vi "Harv_2_9.vi"(0 "HarvSetpoints":dbl[](array[numeric]), 1 "HarvPot":dbl, 3 "Count":i32, 4 "BallAcquired":bool, 5 "FireBallSen":bool, 6 "Fire":bool, 7 "Harvest":bool, 8 "HPButton":bool, 9 "inAuton?":bool, 10 "WinchDown":bool, 11 "AutonMoved":bool, 12 "HarvPivUP":bool, 13 "HarvPivPickupLim":bool) -> (14 "HarvPower":dbl, 15 "HarvRoller":dbl, 16 "AutonReadyToMove":bool, 17 "CountOut":i32, 18 "HarvStart":bool, 19 "HarvCleared":bool)   [LabVIEW 2013]
panel:
  in  "MotorScale":dbl=1.5
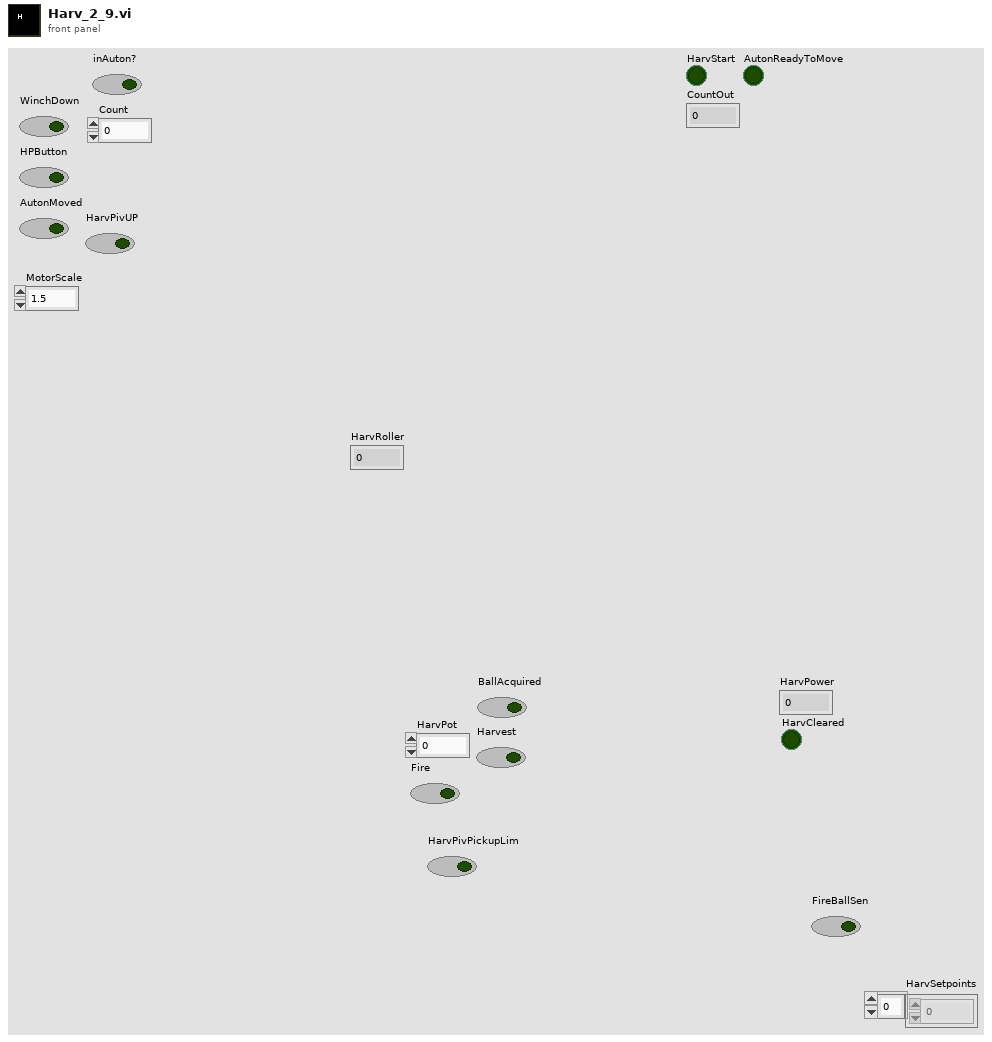
[diagram p1: front panel]
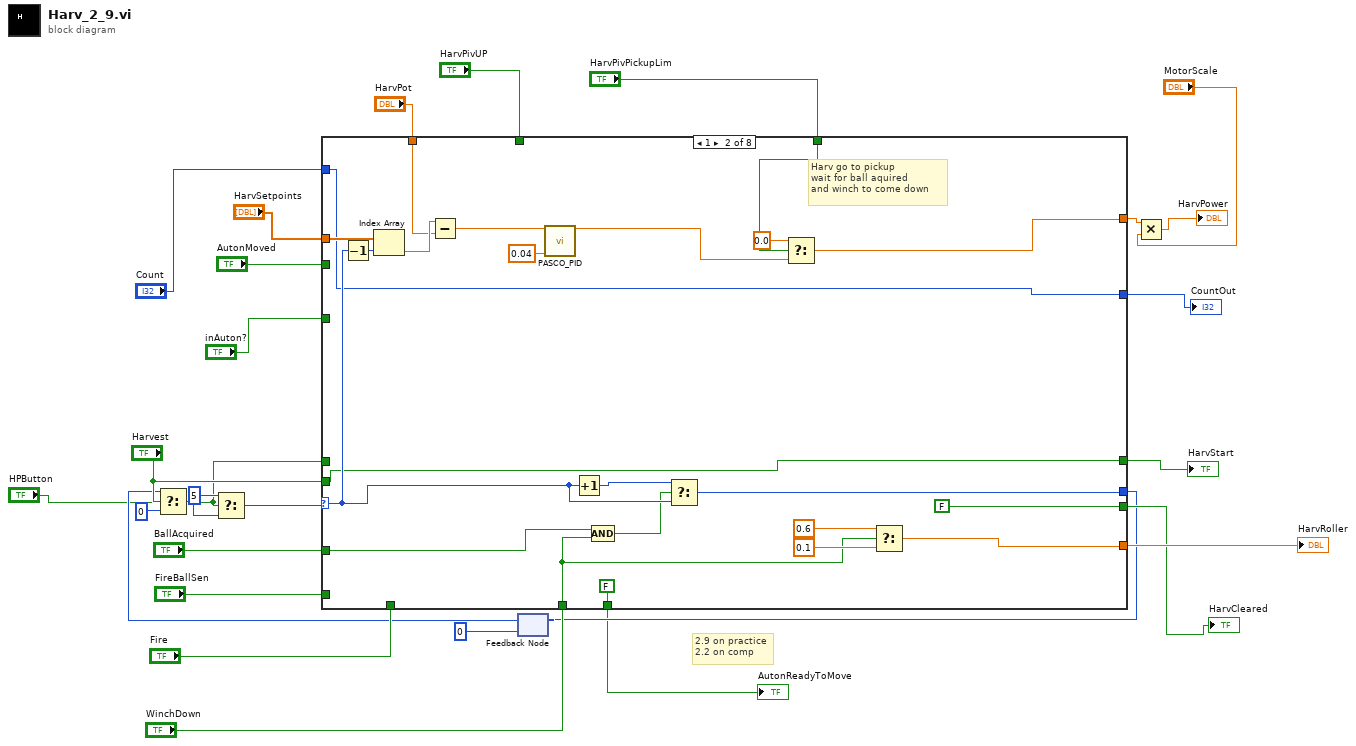
[diagram p0: block diagram]
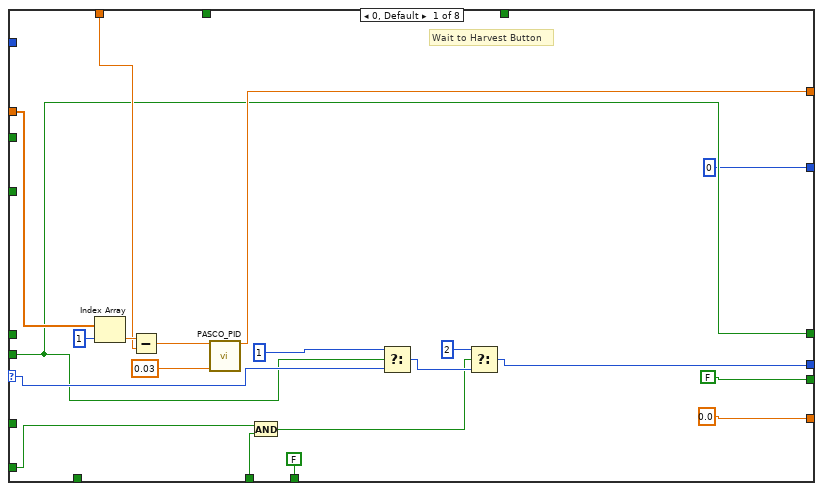
[diagram p2: hidden frame]
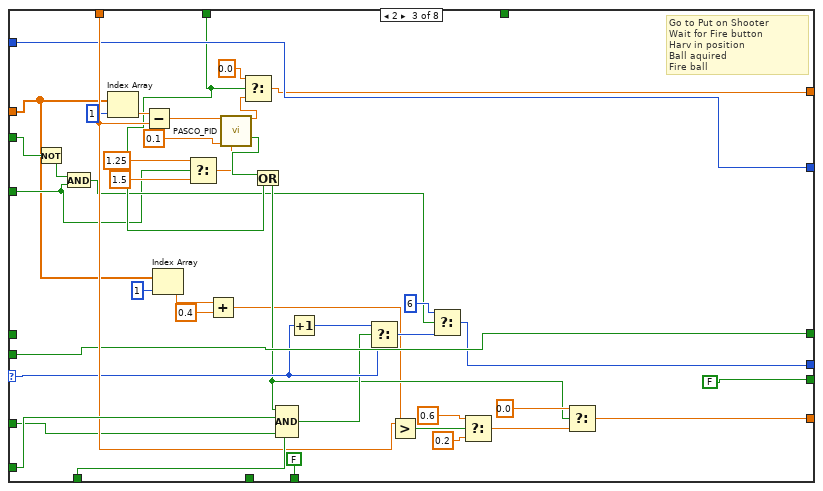
[diagram p3: hidden frame]
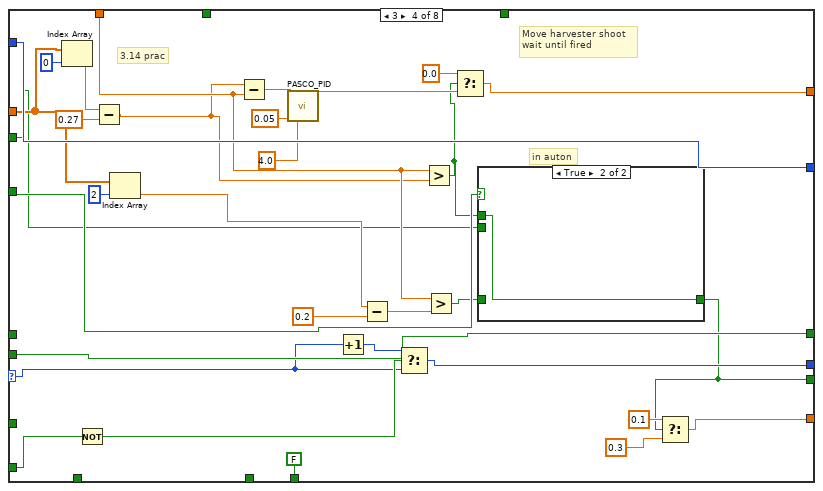
[diagram p4: hidden frame]
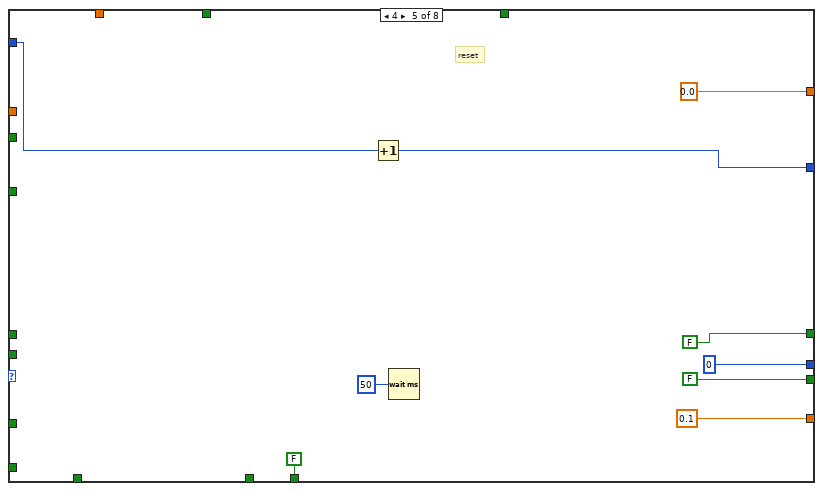
[diagram p6: hidden frame]
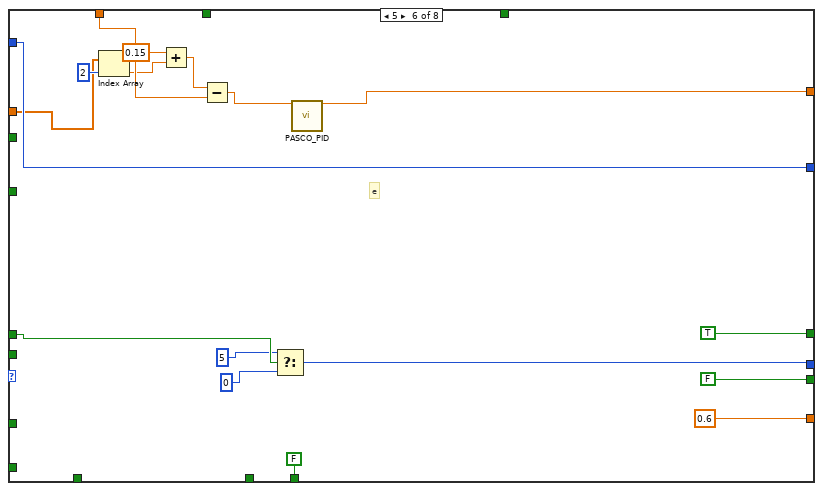
[diagram p7: hidden frame]
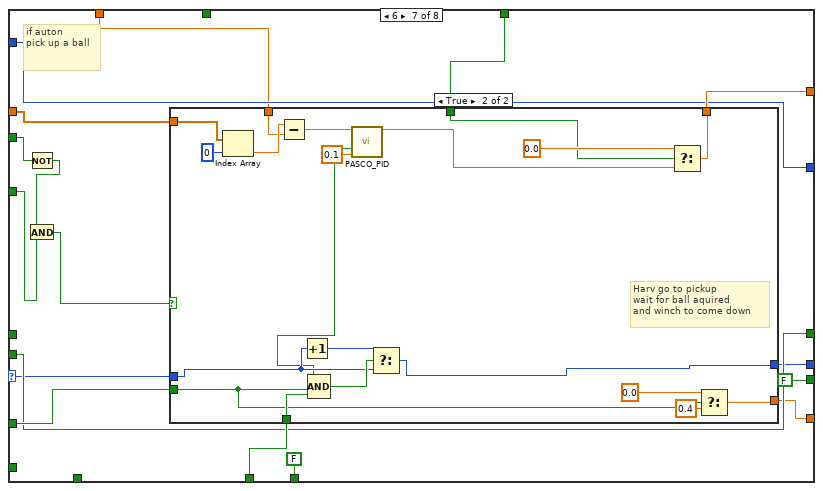
[diagram p8: hidden frame]
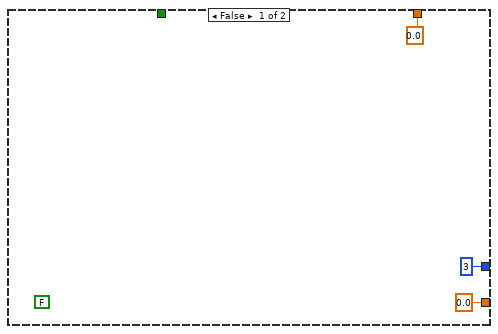
[diagram p9: hidden frame]
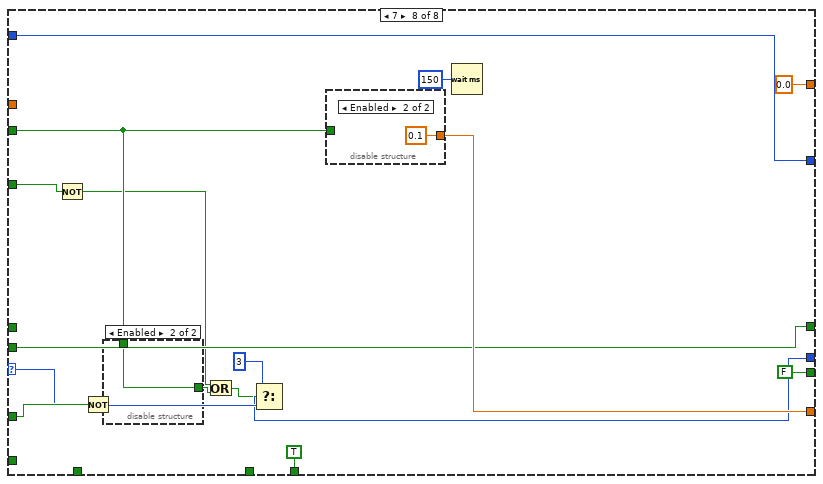
[diagram p10: hidden frame]
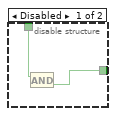
[diagram p11: hidden frame]
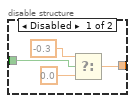
[diagram p12: hidden frame]
diagram:
  # "2.9 on practice\n2.2 on comp"
  n1 = feedback #1(0 ("f")) -> (w21:i32)
  n2 = Select(t=w21, s="Harvest", f=0) -> (s? t:f=w6:i32)
  n3 = Select(t=5, s="HPButton", f=w6) -> (s? t:f=w5:i32)
  n4 = case shown="1" w5 {
    selector: w5 -> [w45 w64 w97 w139 _ _ w182 w223]
    tunnel: "HarvSetpoints" -> [w44 w71 w76 w126 _ w160 w189 _]
    tunnel: "HarvPot" -> [w43 w69 w108 w131 _ w172 w176 _]
    tunnel: [w38 w51 w87 w132 0.0 ("Output") w170 w188 0.0 ("Output")] -> w20
    tunnel: [w35 w66 w89 w144 0 ("t") w165 w183 w222] -> w10
    tunnel: [0.0 ("f") w58 w102 w117 0.1 ("f") 0.6 ("f") w184 w226] -> w26
    tunnel: "BallAcquired" -> [_ w60 w99 _ _ _ w186 w224]
    tunnel: "FireBallSen" -> [w33 _ w111 w142 _ _ _ _]
    tunnel: "Fire" -> [_ _ w110 _ _ _ _ _]
    tunnel: "Harvest" -> [w36 w61 w100 w143 _ _ w185 w225]
    tunnel: [FALSE ("IsThere") FALSE ("IsThere") FALSE ("IsThere") w114 FALSE ("IsThere") FALSE ("IsThere") FALSE ("IsThere") FALSE ("IsThere")] -> w17
    tunnel: "HarvPivPickupLim" -> [_ w53 _ _ _ _ w190 _]
    tunnel: "HarvPivUP" -> [_ _ w92 _ _ _ _ _]
    tunnel: [w36 w61 w100 w143 FALSE ("Harvest") TRUE ("Harvest") w185 w225] -> w14
    tunnel: "WinchDown" -> [w32 w55 _ _ _ _ w187 _]
    tunnel: "inAuton?" -> [_ _ w78 w121 _ _ w177 w215]
    tunnel: [0 ("Count") w54 w96 w138 w150 w169 w181 w228] -> w8
    tunnel: "Count" -> [_ w54 w96 w138 w149 w169 w181 w228]
    tunnel: "HPButton" -> [_ _ _ _ _ w168 _ _]
    tunnel: [FALSE FALSE FALSE FALSE FALSE FALSE FALSE TRUE] -> w2
    tunnel: "AutonMoved" -> [_ _ w84 w118 _ _ w175 w218]
    frame 0, Default {
      # "Wait to Harvest Button"
      n5 = Index Array(array=w44, index=1) -> (element=w46:dbl)
      n6 = Subtract(x=w46, y=w43) -> (x-y=w47:dbl)
      n7 = call "PASCO_PID.vi"("Delta"=w47, "Deadband"=0.03) -> ("Output"=w38:dbl)  [unwired: 12 in, 1 out]
      n8 = And(x=w33, y=w32) -> (x .and. y?=w31:bool)
      n9 = Select(t=1, s=w36, f=w45) -> (s? t:f=w37:i32)
      n10 = Select(t=2, s=w31, f=w37) -> (s? t:f=w35:i32)
    }
    frame 1 {
      # "Harv go to pickup\nwait for ball aquired\nand winch to come down"
      n11 = Decrement(x=w64) -> (x-1=w65:i32)
      n12 = Index Array(array=w71, index=w65) -> (element=w70:dbl)
      n13 = Subtract(x=w70, y=w69) -> (x-y=w68:dbl)
      n14 = call "PASCO_PID.vi"("Delta"=w68, "Deadband"=0.04) -> ("Output"=w52:dbl)  [unwired: 12 in, 1 out]
      n15 = Increment(x=w64) -> (x+1=w67:i32)
      n16 = Compound Arithmetic op=AND(w60, w55) -> (w59:bool)
      n17 = Select(t=w67, s=w59, f=w64) -> (s? t:f=w66:i32)
      n18 = Select(t=0.0, s=w53, f=w52) -> (s? t:f=w51:dbl)
      n19 = Select(t=0.6, s=w55, f=0.1) -> (s? t:f=w58:dbl)
    }
    frame 2 {
      # "Go to Put on Shooter\nWait for Fire button\nHarv in position\nBall aquired \nFire ball"
      n20 = Not(x=w84) -> (.not. x?=w83:bool)
      n21 = And(x=w83, y=w78) -> (x .and. y?=w82:bool)
      n22 = Index Array(array=w76, index=1) -> (element=w113:dbl)
      n23 = Subtract(x=w113, y=w108) -> (x-y=w112:dbl)
      n24 = Index Array(array=w76, index=1) -> (element=w74:dbl)
      n25 = Select(t=1.25, s=w78, f=1.5) -> (s? t:f=w81:dbl)
      n26 = Add(x=w74, y=0.4) -> (x+y=w72:dbl)
      n27 = call "PASCO_PID.vi"("Delta"=w112, "Deadband"=0.1, "P Gain"=w81) -> ("Output"=w95:dbl, "IsThere"=w93:bool)  [unwired: 11 in]
      n28 = Select(t=0.0, s=w92, f=w95) -> (s? t:f=w87:dbl)
      n29 = Or(x=w93, y=w92) -> (x .or. y?=w85:bool)
      n30 = Compound Arithmetic op=AND(w85, w111, w110, w99) -> (w86:bool)
      n31 = Increment(x=w97) -> (x+1=w98:i32)
      n32 = Select(t=w98, s=w86, f=w97) -> (s? t:f=w90:i32)
      n33 = Greater?(x=w108, y=w72) -> (0:w107:bool)
      n34 = Select(t=6, s=w82, f=w90) -> (s? t:f=w89:i32)
      n35 = Select(t=0.6, s=w107, f=0.2) -> (s? t:f=w103:dbl)
      n36 = Select(t=0.0, s=w85, f=w103) -> (s? t:f=w102:dbl)
    }
    frame 3 {
      # "in auton"
      # "3.14 prac"
      # "Move harvester shoot\nwait until fired"
      n37 = Index Array(array=w126, index=0) -> (element=w125:dbl)
      n38 = Not(x=w142) -> (.not. x?=w141:bool)
      n39 = Subtract(x=w125, y=0.27) -> (x-y=w124:dbl)
      n40 = Index Array(array=w126, index=2) -> (element=w129:dbl)
      n41 = Subtract(x=w124, y=w131) -> (x-y=w137:dbl)
      n42 = call "PASCO_PID.vi"("Delta"=w137, "Deadband"=0.05, "P Gain"=4.0) -> ("Output"=w133:dbl)  [unwired: 11 in, 1 out]
      n43 = Increment(x=w139) -> (x+1=w140:i32)
      n44 = Subtract(x=w129, y=0.2) -> (x-y=w130:dbl)
      n45 = Select(t=w140, s=w141, f=w139) -> (s? t:f=w144:i32)
      n46 = Greater?(x=w131, y=w124) -> (0:w119:bool)
      n47 = Greater?(x=w131, y=w130) -> (0:w120:bool)
      n48 = Select(t=0.0, s=w119, f=w133) -> (s? t:f=w132:dbl)
      n49 = case shown="True" w121 {
        tunnel: [w146 w147] -> w114
        tunnel: w120 -> [w146 _]
        tunnel: w119 -> [_ w147]
        tunnel: w118 -> [_ _]
        frame False {
        }
        frame True {
        }
      }
      n50 = Select(t=0.1, s=w114, f=0.3) -> (s? t:f=w117:dbl)
    }
    frame 4 {
      # "reset"
      n51 = Increment(x=w149) -> (x+1=w150:i32)
      n52 = Wait (ms)(milliseconds to wait=u32 50) -> ()  [unwired: 1 out]
    }
    frame 5 {
      # "e"
      n53 = Index Array(array=w160, index=2) -> (element=w158:dbl)
      n54 = Add(x=0.15, y=w158) -> (x+y=w157:dbl)
      n55 = Subtract(x=w157, y=w172) -> (x-y=w171:dbl)
      n56 = Select(t=5 ("index"), s=w168, f=0 ("index")) -> (s? t:f=w165:i32)
      n57 = call "PASCO_PID.vi"("Delta"=w171) -> ("Output"=w170:dbl)  [unwired: 13 in, 1 out]
    }
    frame 6 {
      # "if auton \npick up a ball"
      n58 = Not(x=w175) -> (.not. x?=w174:bool)
      n59 = And(x=w174, y=w177) -> (x .and. y?=w178:bool)
      n60 = case shown="True" w178 {
        tunnel: w190 -> [_ w209]
        tunnel: w189 -> [_ w208]
        tunnel: [0.0 ("Output") w206] -> w188
        tunnel: w187 -> [_ w205]
        tunnel: w186 -> [_ w203]
        tunnel: [0.0 ("f") w204] -> w184
        tunnel: [3 w199] -> w183
        tunnel: w182 -> [_ w197]
        tunnel: w176 -> [_ w195]
        frame False {
          (unwired) FALSE
        }
        frame True {
          # "Harv go to pickup\nwait for ball aquired\nand winch to come down"
          n61 = Index Array(array=w208, index=0) -> (element=w196:dbl)
          n62 = Subtract(x=w196, y=w195) -> (x-y=w210:dbl)
          n63 = Increment(x=w197) -> (x+1=w198:i32)
          n64 = call "PASCO_PID.vi"("Delta"=w210, "Deadband"=0.1) -> ("Output"=w212:dbl, "IsThere"=w194:bool)  [unwired: 12 in]
          n65 = Compound Arithmetic op=AND(w194, w203, w205) -> (w200:bool)
          n66 = Select(t=w198, s=w200, f=w197) -> (s? t:f=w199:i32)
          n67 = Select(t=0.0, s=w209, f=w212) -> (s? t:f=w206:dbl)
          n68 = Select(t=0.0, s=w203, f=0.4) -> (s? t:f=w204:dbl)
        }
      }
    }
    frame 7 {
      n69 = Not(x=w215) -> (.not. x?=w214:bool)
      n70 = Not(x=w224) -> ()  [unwired: 1 out]
      n71 = disable-structure shown="Enabled" {
        disable-tunnel: w218 -> [w232 w233]
        disable-tunnel: [w231 w233] -> w216
        frame Disabled {
          n72 = And(x=w232, y=w231) -> (x .and. y?=w230:bool)
        }
        frame Enabled {
        }
      }
      n73 = Or(x=w214, y=w216) -> (x .or. y?=w217:bool)
      n74 = Select(t=3, s=w217, f=w223) -> (s? t:f=w222:i32)
      n75 = disable-structure shown="Enabled" {
        disable-tunnel: [w237 0.1 ("f")] -> w226
        disable-tunnel: w218 -> [w234 _]
        frame Disabled {
          n76 = Select(t=-0.3, s=w234, f=0.0) -> (s? t:f=w237:dbl)
        }
        frame Enabled {
        }
      }
      n77 = Wait (ms)(milliseconds to wait=u32 150) -> ()  [unwired: 1 out]
    }
  }
  "HarvRoller" <- w26
  "HarvCleared" <- w17
  "HarvStart" <- w14
  "CountOut" <- w8
  "AutonReadyToMove" <- w2
  n78 = feedback-in #1(w10) -> ()
  n79 = Multiply(x=w20, y="MotorScale") -> (x*y=→"HarvPower":dbl)
